vi "Initialisation_Emballage_BDD.vi"(11 "entrée d'erreur (pas d'erreur)":errorcluster) -> (8 "Produits_Commandes_en_cours.txt":path, 10 "Tab codif-code bar":string[][](array[string]), 15 "sortie d'erreur":errorcluster)   [LabVIEW 2020]
uses:
  Modules/FS/60_FS_Controles/60_FS_SetGet.ctl
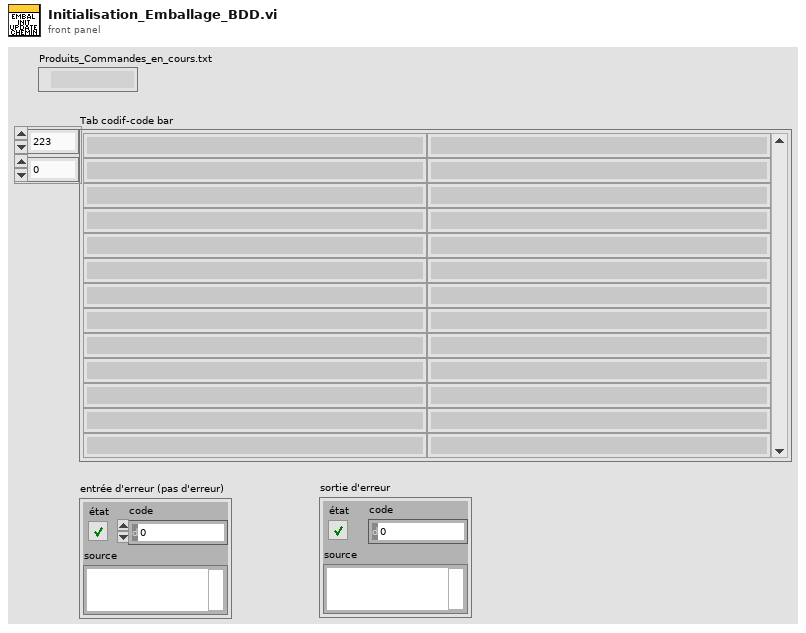
[diagram p1: front panel]
types:
  T1 = typedef "60_FS_SetGet.ctl" = enum16{"set", "get"}
  T2 = cluster{"Admin-réseau":path, "XML-Réseau":path, " Résultat tests-Réseau":path, " Archive prôbleme-Réseau":path, " Archive Test  Local":path}
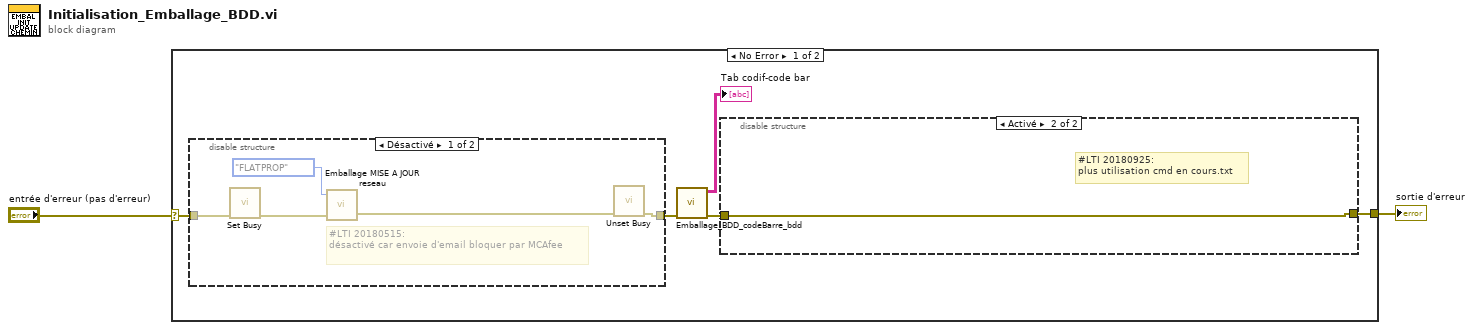
[diagram p0: block diagram]
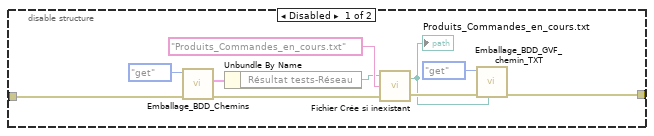
[diagram p2: hidden frame]
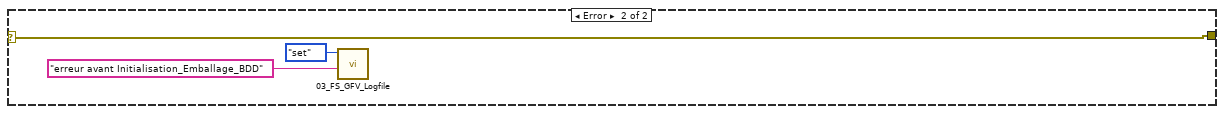
[diagram p4: hidden frame]
diagram:
  n1 = case shown="No Error" "entrée d'erreur (pas d'erreur)" {
    selector: "entrée d'erreur (pas d'erreur)" -> [w5 w27]
    tunnel: [w3 w27] -> w1
    frame No Error {
      n2 = disable-structure shown="Désactivé" {
        disable-tunnel: [w23 w24] -> w7
        disable-tunnel: w5 -> [w19 w24]
        frame Disabled {
          # "#LTI 20180515:\ndésactivé car envoie d'email bloquer par MCAfee"
          n3 = call <vilib>:"Set Busy.vi"("error in (no error)"=w19) -> ("error out"=w21:errorcluster)  [unwired: 9 in, 1 out]
          n4 = call "Emballage MISE A JOUR reseau.vi"("error in (no error)"=w21, "DIVISION"=enum16{"FLATPROP", "MEDIC"}."FLATPROP") -> ("error out"=w22:errorcluster)  [unwired: 3 in]
          n5 = call <vilib>:"Unset Busy.vi"("error in (no error)"=w22) -> ("error out"=w23:errorcluster)  [unwired: 10 in]
        }
        frame Enabled {
        }
      }
      n6 = call "Emballage_BDD_codeBarre_bdd.vi"("Error in"=w7) -> ("Error out"=w4:errorcluster, "tableau ajouté"=→"Tab codif-code bar":string[][])  [unwired: 9 in]
      n7 = disable-structure shown="Activé" {
        disable-tunnel: w4 -> [w13 w18]
        disable-tunnel: [w9 w18] -> w3
        frame Disabled {
          n8 = call "Emballage_BDD_Chemins.vi"("error in (no error)"=w13, "SetGet"=60_FS_SetGet."get") -> ("error out"=w12:errorcluster, "CLT_Chemins_out"=w16:T2)  [unwired: 8 in]
          n9 = Unbundle By Name(w16) -> ("Résultat tests-Réseau"=w14:path)
          n10 = call "Fichier Crée si inexistant.vi"("error in"=w12, "nom fichier"="Produits_Commandes_en_cours.txt", "chemin du dossier IN"=w14) -> ("error out"=w10:errorcluster, "chemin sous dossier OUT"=w8:path)
          "Produits_Commandes_en_cours.txt" <- w8
          n11 = call "Emballage_BDD_GVF_chemin_TXT.vi"("Produits_Commandes_en_cours.txt IN"=w8, "Error in"=w10, "Énum"=enum16{"get", "set"}."get") -> ("Error out"=w9:errorcluster)  [unwired: 7 in, 1 out]
        }
        frame Enabled {
          # "#LTI 20180925:\nplus utilisation cmd en cours.txt"
        }
      }
    }
    frame Error {
      n12 = call "03_FS_GFV_Logfile.vi"("Chaîne"="erreur avant Initialisation_Emballage_BDD", "States"=60_FS_SetGet."set") -> ()  [unwired: 8 in, 2 out]
    }
  }
  "sortie d'erreur" <- w1
